vi "GOMDBTS2048 substitution Geo Set Dynamic Time Mode.vi"(8 "error in (no error)":errorcluster, 10 "value":bool, 11 "handle":i32) -> (0 "error out":errorcluster, 3 "function return":i32)   [LabVIEW 2015, in "GOMDBTS2048.lvlib"]
doc: "GOBTS2048DLL int __stdcall GOMDBTS2048_substitutionSetIntegrationTimeInUs(int handle, int value);"
uses:
  GOMDBTS2048.lvlib
  runtime/GOMDBTS2048.dll
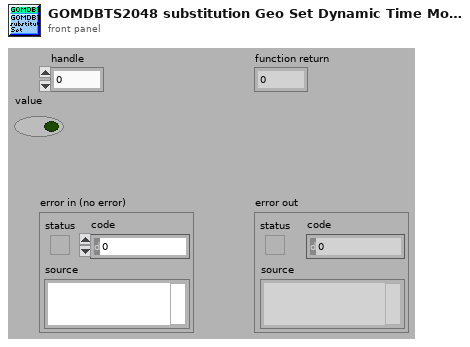
[diagram p1: front panel]
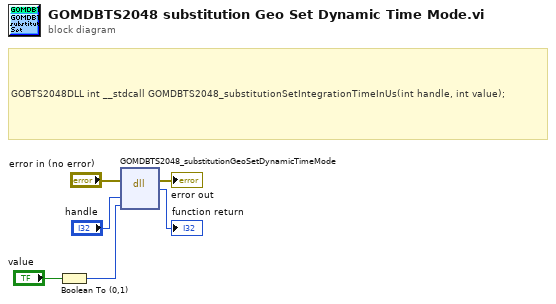
[diagram p0: block diagram]
diagram:
  # "GOBTS2048DLL int __stdcall GOMDBTS2048_substitutionSetIntegrationTimeInUs(int handle, int value);"
  n1 = Boolean To (0,1)(Boolean="value") -> (0, 1=w2:i16)
  n2 = dll-call lib="C:/Users/rkoch/Documents/GO_Library/runtime/GOMDBTS2048.*" fn="GOMDBTS2048_substitutionGeoSetDynamicTimeMode"(error in="error in (no error)", "handle"="handle", "value"=w2) -> (error out=→"error out":errorcluster, "return type"=→"function return":i32)  [unwired: 4 in, 1 out]
